vi "SetVoltage.vi"() -> ()   [LabVIEW 2022 SP3]
uses:
  <instrlib>/Keithley 648X Series/Keithley 648X Series.lvlib
panel:
  in  "Voltage Range":u16(ring) items=["10"=10, "50"=50, "500"=500]
  in  "Current Limit mA":u16
  in  "Voltage":dbl
  in  "Serial Configuration":T1={"Baud Rate"=9600, "Parity"=0, "Data Bits"=8, "Stop Bits"=10, "Flow Control"=0} {"Flow Control" items=["None", "XON/XOFF", "RTS/CTS", "XON/XOFF & RTS/CTS", "DTR/DSR", "XON/XOFF & DTR/DSR"]; "Stop Bits" items=["1.0"=10, "1.5"=15, "2.0"=20]; "Data Bits" items=["7"=7, "8"=8]; "Parity" items=["None", "Odd", "Even", "Mark", "Space"]; "Baud Rate" items=["300"=300, "600"=600, "1200"=1200, "2400"=2400, "4800"=4800, "9600"=9600, "19200"=19200]}
  in  "VISA resource name":refnum<visa-resource-name>
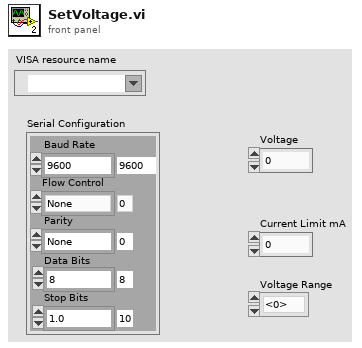
[diagram p1: front panel]
types:
  T1 = cluster{"Baud Rate":u32, "Parity":u16, "Data Bits":u16, "Stop Bits":u16, "Flow Control":u16}
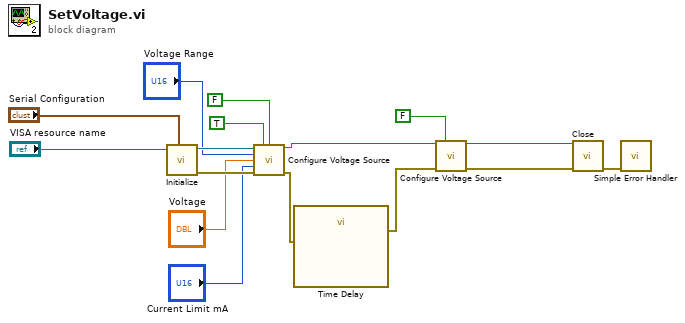
[diagram p0: block diagram]
diagram:
  n1 = call <instrlib>:"Initialize.vi"("Serial Configuration"="Serial Configuration", "VISA resource name"="VISA resource name") -> ("error out"=w13:errorcluster, "VISA resource name out"=w14:refnum<visa-resource-name>)  [unwired: 8 in]
  n2 = call <instrlib>:"Configure Voltage Source.vi"("VISA resource name"=w14, "Enable Voltage Source (F: Disable)"=TRUE, "Enable Interlock (F: Disable)"=FALSE, "Voltage Source Range (10 V)"="Voltage Range", "Voltage Level (0 V)"="Voltage", "Current Limit (25 mA)"="Current Limit mA", "error in (no error)"=w13) -> ("VISA resource name out"=w6:refnum<visa-resource-name>, "error out"=w7:errorcluster)  [unwired: 7 in]
  n3 = call "Time Delay"("error in (no error)"=w7) -> ("error out"=w5:errorcluster)  [unwired: 10 in]
  n4 = call <instrlib>:"Configure Voltage Source.vi"("VISA resource name"=w6, "Enable Voltage Source (F: Disable)"=FALSE, "error in (no error)"=w5) -> ("VISA resource name out"=w3:refnum<visa-resource-name>, "error out"=w4:errorcluster)  [unwired: 11 in]
  n5 = call <instrlib>:"Close.vi"("error in (no error)"=w4, "VISA resource name"=w3) -> ("error out"=w1:errorcluster)  [unwired: 9 in]
  n6 = call <vilib>:"Simple Error Handler.vi"("error in (no error)"=w1) -> ()  [unwired: 4 in, 5 out]
